vi "UDP_Read_bool.vi"() -> ()   [LabVIEW 2014]
panel:
  out "Boolean":bool
  in  "stop":bool
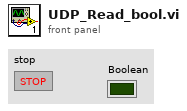
[diagram p1: front panel]
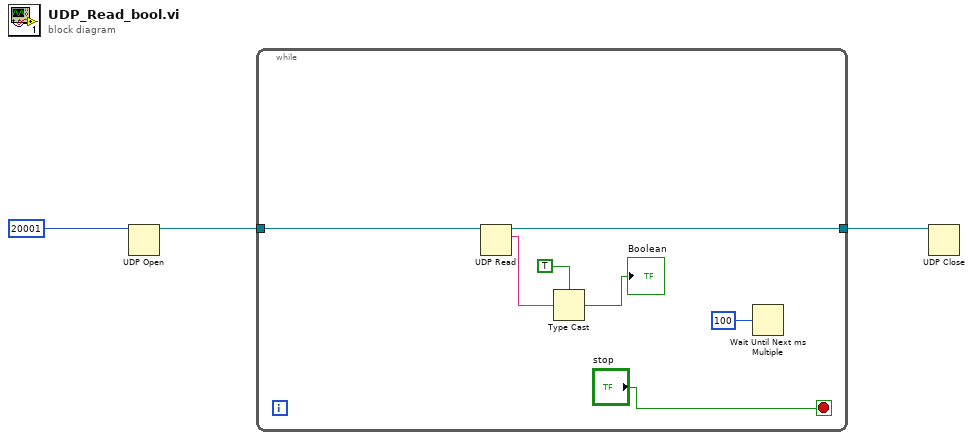
[diagram p0: block diagram]
diagram:
  n1 = UDP Open(11:u16 20001 ("port")) -> (port=w2:refnum<k16>)  [unwired: 4 in, 2 out]
  n2 = while {
    tunnel: w2 -> [w10]
    tunnel: [w9] -> w1
    stop <- "stop" stop-if-true
    n3 = UDP Read(connection ID=w10) -> (data out=w6:string, 3:w9:refnum<k16>)  [unwired: 3 in, 3 out]
    n4 = Type Cast(type=TRUE, x=w6) -> (*(type *) &x=→"Boolean":bool)
    n5 = Wait Until Next ms Multiple(millisecond multiple=u32 100) -> ()  [unwired: 1 out]
  }
  n6 = UDP Close(connection ID=w1) -> ()  [unwired: 1 in, 2 out]
